vi "Check Lock.vi"(8 "error in (no error)":errorcluster, 9 "Control level":T1, 10 "Name":string, 11 "BME_DG_System in":refnum<class "BME_DG_System.lvclass">) -> (0 "error out":errorcluster, 1 "Control level out":T1, 2 "Locked by":string, 3 "BME_DG_System out":refnum<class "BME_DG_System.lvclass">, 5 "Ok?":bool)   [LabVIEW 2009, in "POLARIS BME DG.lvlib" / "BME_DG_System.lvclass"]
uses:
  BME_DG_System.lvclass
  ControlLevel.ctl
  BME_DG_System.lvclass/BME_DG_System.ctl
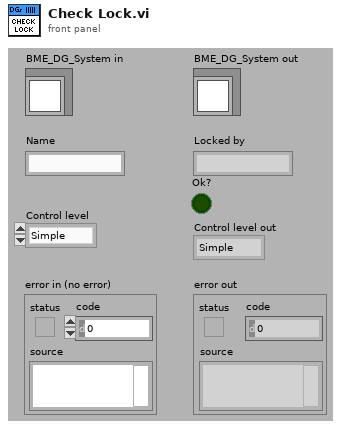
[diagram p1: front panel]
types:
  T1 = typedef "POLARIS BME DG.lvlib/BME_DG_System.lvclass/ControlLevel.ctl" = enum16{"Simple", "Expert", "Unknown"}
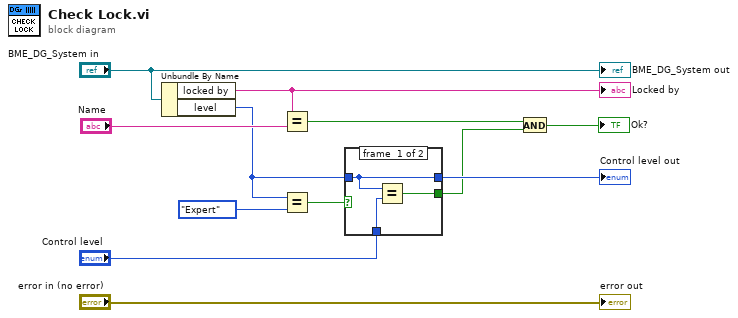
[diagram p0: block diagram]
diagram:
  n1 = Unbundle By Name("BME_DG_System in") -> ("locked by"=w7:string, "level"=w3:T1)
  "Locked by" <- w7
  n2 = Equal?(x=w7, y="Name") -> (x = y?=w1:bool)
  n3 = Equal?(x=w3, y=ControlLevel."Expert" ("Control level 2")) -> (x = y?=w4:bool)
  n4 = case shown="False" w4 {
    selector: w4 -> [_ w17]
    tunnel: w3 -> [w13 w16]
    tunnel: "Control level" -> [w15 _]
    tunnel: [w14 w17] -> w2
    tunnel: [w13 w16] -> w6
    frame #0 {
      n5 = Equal?(x=w13, y=w15) -> (x = y?=w14:bool)
    }
    frame #1 {
    }
  }
  "Control level out" <- w6
  n6 = And(x=w1, y=w2) -> (x .and. y?=→"Ok?":bool)
  "error out" <- "error in (no error)"
  "BME_DG_System out" <- "BME_DG_System in"
